vi "numeric operations 3.vi"() -> ()   [LabVIEW 2020]
panel:
  out "volume":dbl
  in  "height":dbl
  in  "radius":dbl
  out "volume":dbl
  in  "radius":dbl
  out "cube":dbl
  in  "number":dbl
  in  "height":dbl
  out "volume":dbl
  in  "radius":dbl
  out "circumference":dbl
  in  "radius":dbl
  out "Boolean 2":bool
  in  "Boolean":bool
  in  "Tab Control":enum32{"Page 1", "Page 2"}(tab)
  in  "radius 2":dbl(knob) scale=0.0..10.0
  out "circumference 2":dbl(knob) scale=0.0..100.0
  # "circumference"
  # "volume of cylinder"
  # "cube"
  # "volume of sphere"
  # "volume of cone"
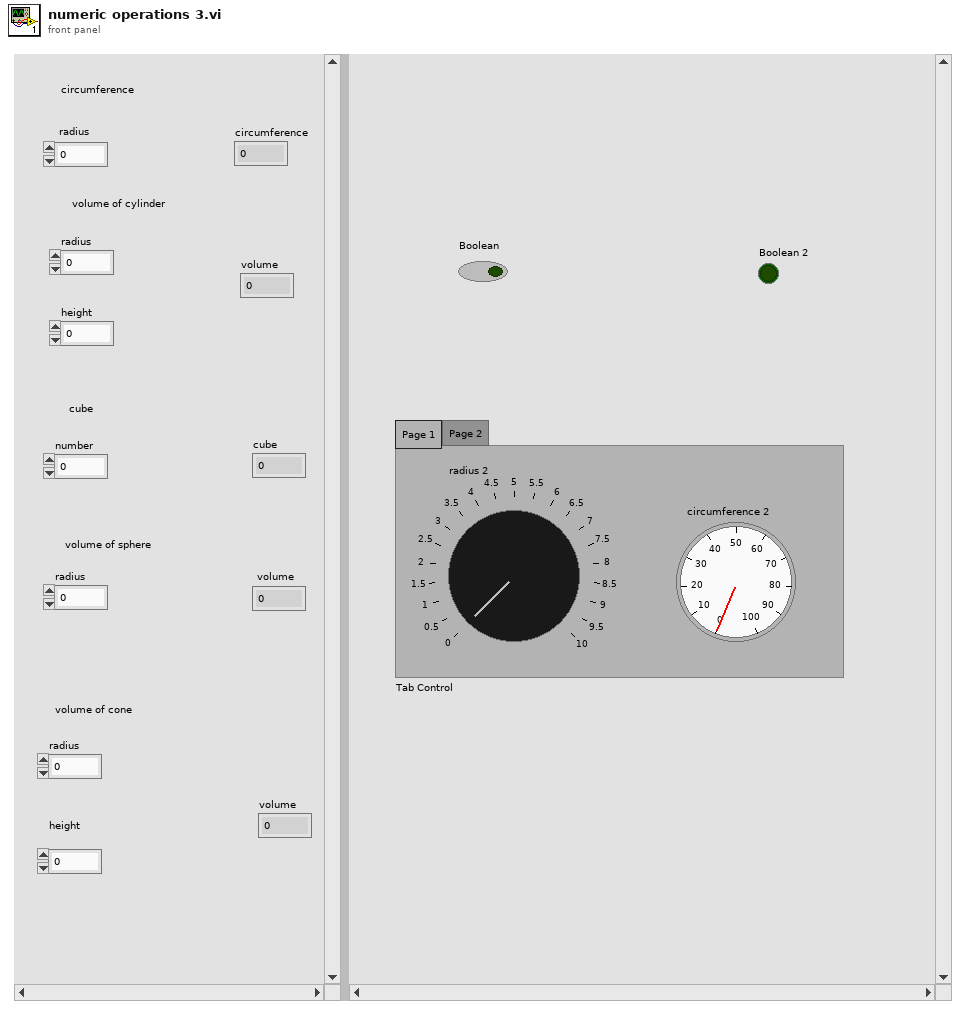
[diagram p1: front panel]
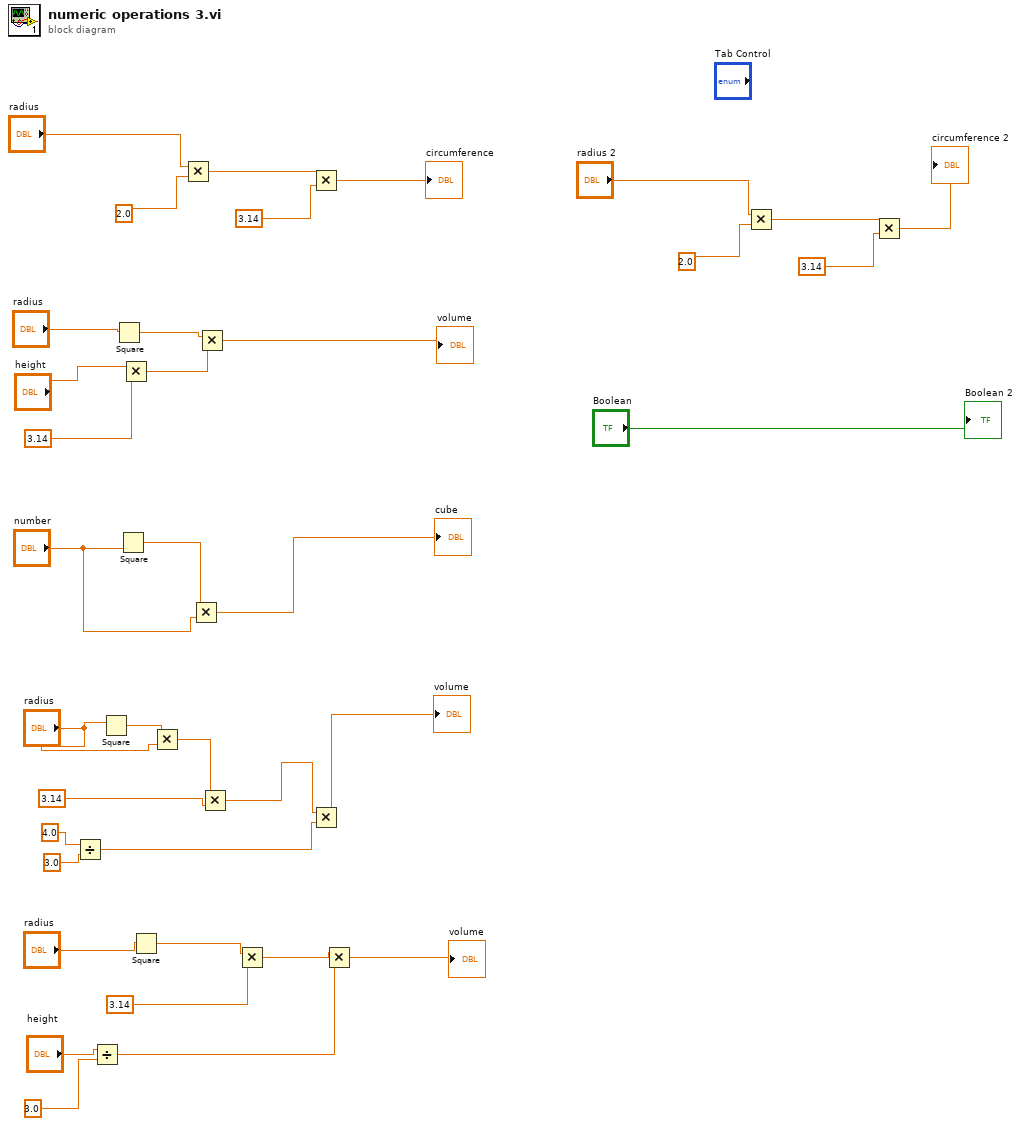
[diagram p0: block diagram]
diagram:
  n1 = Divide(x=4.0, y=3.0) -> (x/y=w16:dbl)
  n2 = Divide(x="height", y=3.0) -> (x/y=w8:dbl)
  n3 = Square(x="radius") -> (x^2=w23:dbl)
  n4 = Square(x="radius") -> (x^2=w31:dbl)
  n5 = Square(x="number") -> (x^2=w26:dbl)
  n6 = Multiply(x="height", y=3.14) -> (x*y=w27:dbl)
  n7 = Square(x="radius") -> (x^2=w11:dbl)
  n8 = Multiply(x=w23, y="radius") -> (x*y=w19:dbl)
  n9 = Multiply(x="radius", y=2.0) -> (x*y=w36:dbl)
  n10 = Multiply(x=w26, y="number") -> (x*y=→"cube":dbl)
  n11 = Multiply(x=w31, y=w27) -> (x*y=→"volume":dbl)
  n12 = Multiply(x=w19, y=3.14) -> (x*y=w17:dbl)
  n13 = Multiply(x=w11, y=3.14) -> (x*y=w9:dbl)
  n14 = Multiply(x=w36, y=3.14) -> (x*y=→"circumference":dbl)
  n15 = Multiply(x=w17, y=w16) -> (x*y=→"volume":dbl)
  n16 = Multiply(x=w9, y=w8) -> (x*y=→"volume":dbl)
  n17 = Multiply(x="radius 2", y=2.0) -> (x*y=w4:dbl)
  n18 = Multiply(x=w4, y=3.14) -> (x*y=→"circumference 2":dbl)
  "Boolean 2" <- "Boolean"
